vi "2_05.vi"() -> ()   [LabVIEW 2018]
uses:
  <vilib>/Analysis/4window.llb/windowTd.ctl
  <vilib>/Analysis/3filter.llb/Filter Passband Type.ctl
  <vilib>/Analysis/1siggen.llb/Ramp Pattern by Samples.vi
  <vilib>/Analysis/2dsp.llb/Real FFT.vi
  <vilib>/Analysis/NI_AALPro.lvlib
  <vilib>/Analysis/NI_AALBase.lvlib
panel:
  out "XY Graph":cluster{dbl[], "Ramp Pattern":dbl[]}(graph)
  in  "filter type":T1=enum."Bandstop"
  in  "Ventana":T2 items=["Rectangle"=0, "Hanning"=1, "Hamming"=2, "Blackman-Harris"=3, "Exact Blackman"=4, "Blackman"=5, "Flat Top"=6, "4 Term B-Harris "=7, "7 Term B-Harris"=8, "Low Sidelobe"=9, "Blackman Nuttall"=11, "Triangle"=30, "Bartlett-Hanning"=31, "Bohman"=32, "Parzen"=33, "Welch"=34, "Kaiser"=60, "Dolph-Chebyshev"=61, "Gaussian"=62]
  in  "Cantidad de Taps":i32=3001 min=1
  in  "Frecuencia de  corte bajo":dbl=950.0 format="%0.2f"
  in  "Frecuencia de corte alto":dbl=1050.0 format="%0.2f"
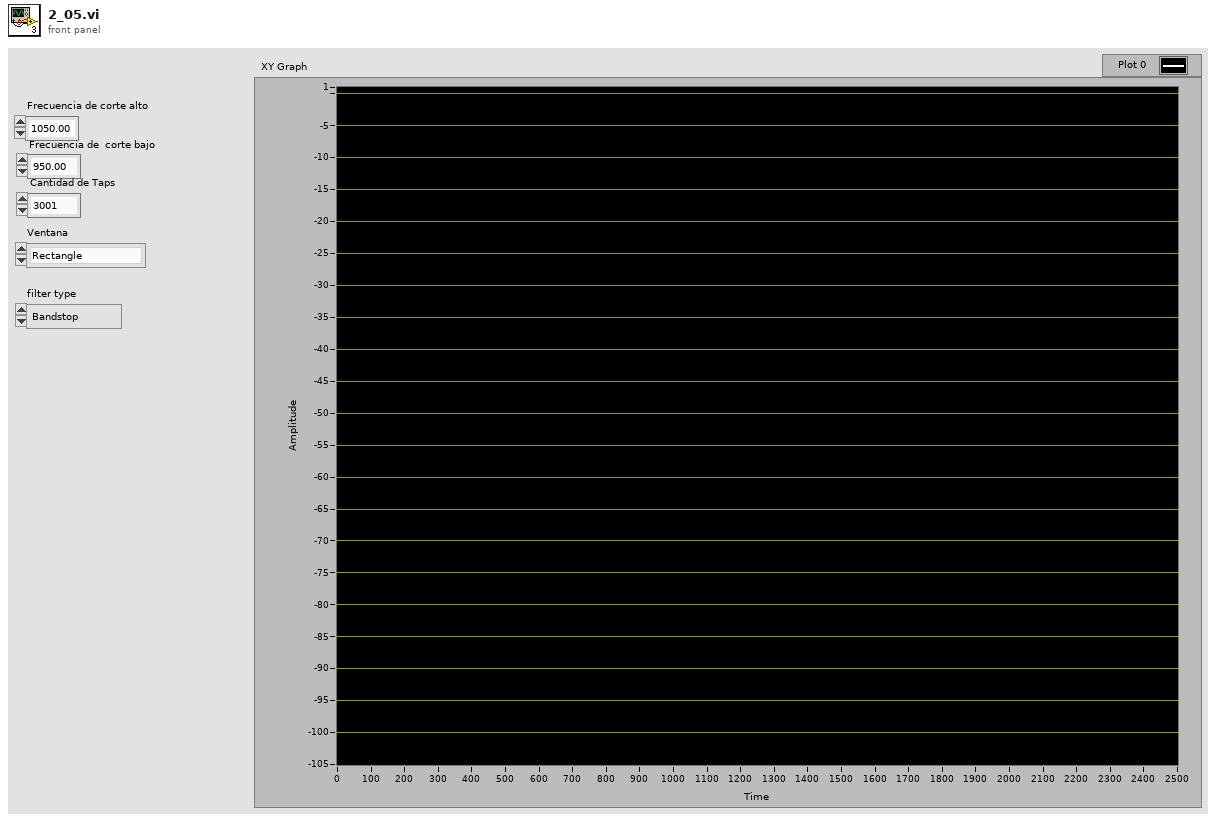
[diagram p1: front panel]
types:
  T1 = typedef "NI_AALBase.lvlib/Filter Passband Type.ctl" = enum32{"Lowpass", "Highpass", "Bandpass", "Bandstop"}
  T2 = typedef "NI_AALPro.lvlib/windowTd.ctl" = u32
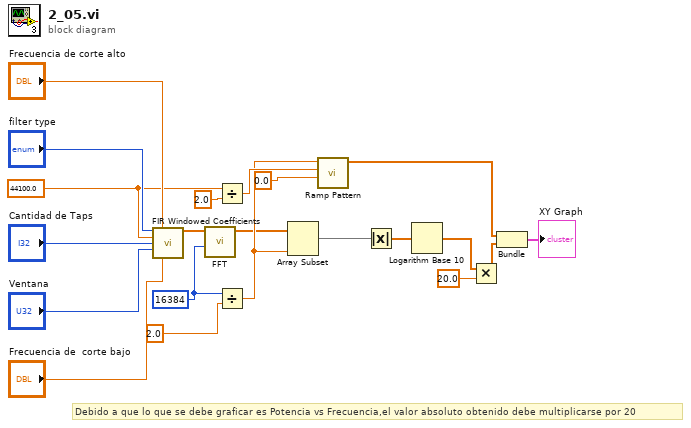
[diagram p0: block diagram]
diagram:
  w5 = 44100.0 ("sampling freq: fs")
  w15 = 16384 ("FFT size")
  # "Debido a que lo que se debe graficar es Potencia vs Frecuencia,el valor absoluto obtenido debe multiplicarse por 20"
  n1 = call <vilib>:"FIR Windowed Coefficients.vi"("filter type"="filter type", "high cutoff freq: fh"="Frecuencia de corte alto", "sampling freq: fs"=w5, "taps"="Cantidad de Taps", "window"="Ventana", "low cutoff freq: fl"="Frecuencia de  corte bajo") -> ("FIR Windowed Coefficients"=w6:dbl[])  [unwired: 8 in, 1 out]
  n2 = call-poly <vilib>:"FFT.vi"("FFT size"=w15, "X"=w6) -> ("FFT {X}"=w13:cdb[])  [unwired: 8 in, 1 out]
  n3 = Divide(x=w5, y=2.0) -> (x/y=w19:dbl)
  n4 = Divide(x=w15, y=2.0) -> (x/y=w14:dbl)
  n5 = Array Subset(array=w13, length=w14) -> (w18:cdb[])  [unwired: 1 in]
  n6 = call-poly <vilib>:"Ramp Pattern.vi"("start"=0.0, "end"=w19, "samples"=w14) -> ("Ramp Pattern"=w12:dbl[])  [unwired: 7 in, 1 out]
  n7 = Absolute Value(x=w18) -> (abs(x)=w17:dbl[])
  n8 = Logarithm Base 10(1:w17) -> (0:w3:dbl[])
  n9 = Multiply(x=w3, y=20.0) -> (x*y=w2:dbl[])
  n10 = Bundle("Ramp Pattern"=w12, w2) -> (→"XY Graph":cluster{"Ramp Pattern":dbl[], dbl[]})  [unwired: 1 in]
